vi "GermanInfo_settings_ut_test.vi"(8 "Error In":errorcluster, 11 "CSMinfo in":T1 {"Окно с настройками"."scheme" items=["NORMAL", "NORMAL_IMMEDIATE_START", "TIMEOUT_T3", "ALLRV_REQ", "SUPPRESS_MSD", "SUPPRESS_ALACK", "SUPPRESS_SEND_MSD"]}) -> (0 "Error Out":errorcluster, 3 "CSMinfo out":T1 {"Окно с настройками"."scheme" items=["NORMAL", "NORMAL_IMMEDIATE_START", "TIMEOUT_T3", "ALLRV_REQ", "SUPPRESS_MSD", "SUPPRESS_ALACK", "SUPPRESS_SEND_MSD"]})   [LabVIEW 2018]
uses:
  MOKO_LabViewLibrary/MokoSTM/MokoClassicUtilitySTM/MCUS_ITEM.ctl
  MOKO_LabViewLibrary/MokoSTM/MokoClassicUtilitySTM/MCUS_STM.ctl
  <vilib>/addons/_JKI.lib/Serialization/JSON/JKI JSON Serialization.lvlib
  GermanInfo.ctl
panel:
  in  "Input attenuation 5":dbl=1.0
  in  "Input attenuation 4":dbl=1.0
  in  "Input attenuation 3":dbl=1.0
  in  "Reset":bool
  in  "Open":bool
  in  "Save":bool
  in  "Setting Path":path
  in  "Применить":bool
  in  "Input attenuation 2":dbl=1.0
  in  "Режим звонка связь":u16(ring) items=["Автоматически (AT) GEMALTO", "Автоматически (AT) SIMCOM", "Автоматически (AT) SIMCOM SIM7600E-H", "Автоматически (AT) TELIT", "Автоматически (AT) PROGRESS", "Автоматически (AT) PROGRESS GREEN", "Автоматически (AT) PROGRESS BLUE", "Автоматически (реле)", "Вручную"]
  # "Входное напряжение (Uin_PS):"
  # "Входной ток (Iin_PS):"
  # "0,4\n0,6\n1\n1,5\n1,6\n2,5\n4"
  # "kPa\nbar\nkgf/cm2\nMPa"
  # "Выходное напряжение (Uout_EL):"
  # "Выходной ток (Iout_EL):"
  # "Схема измерений:"
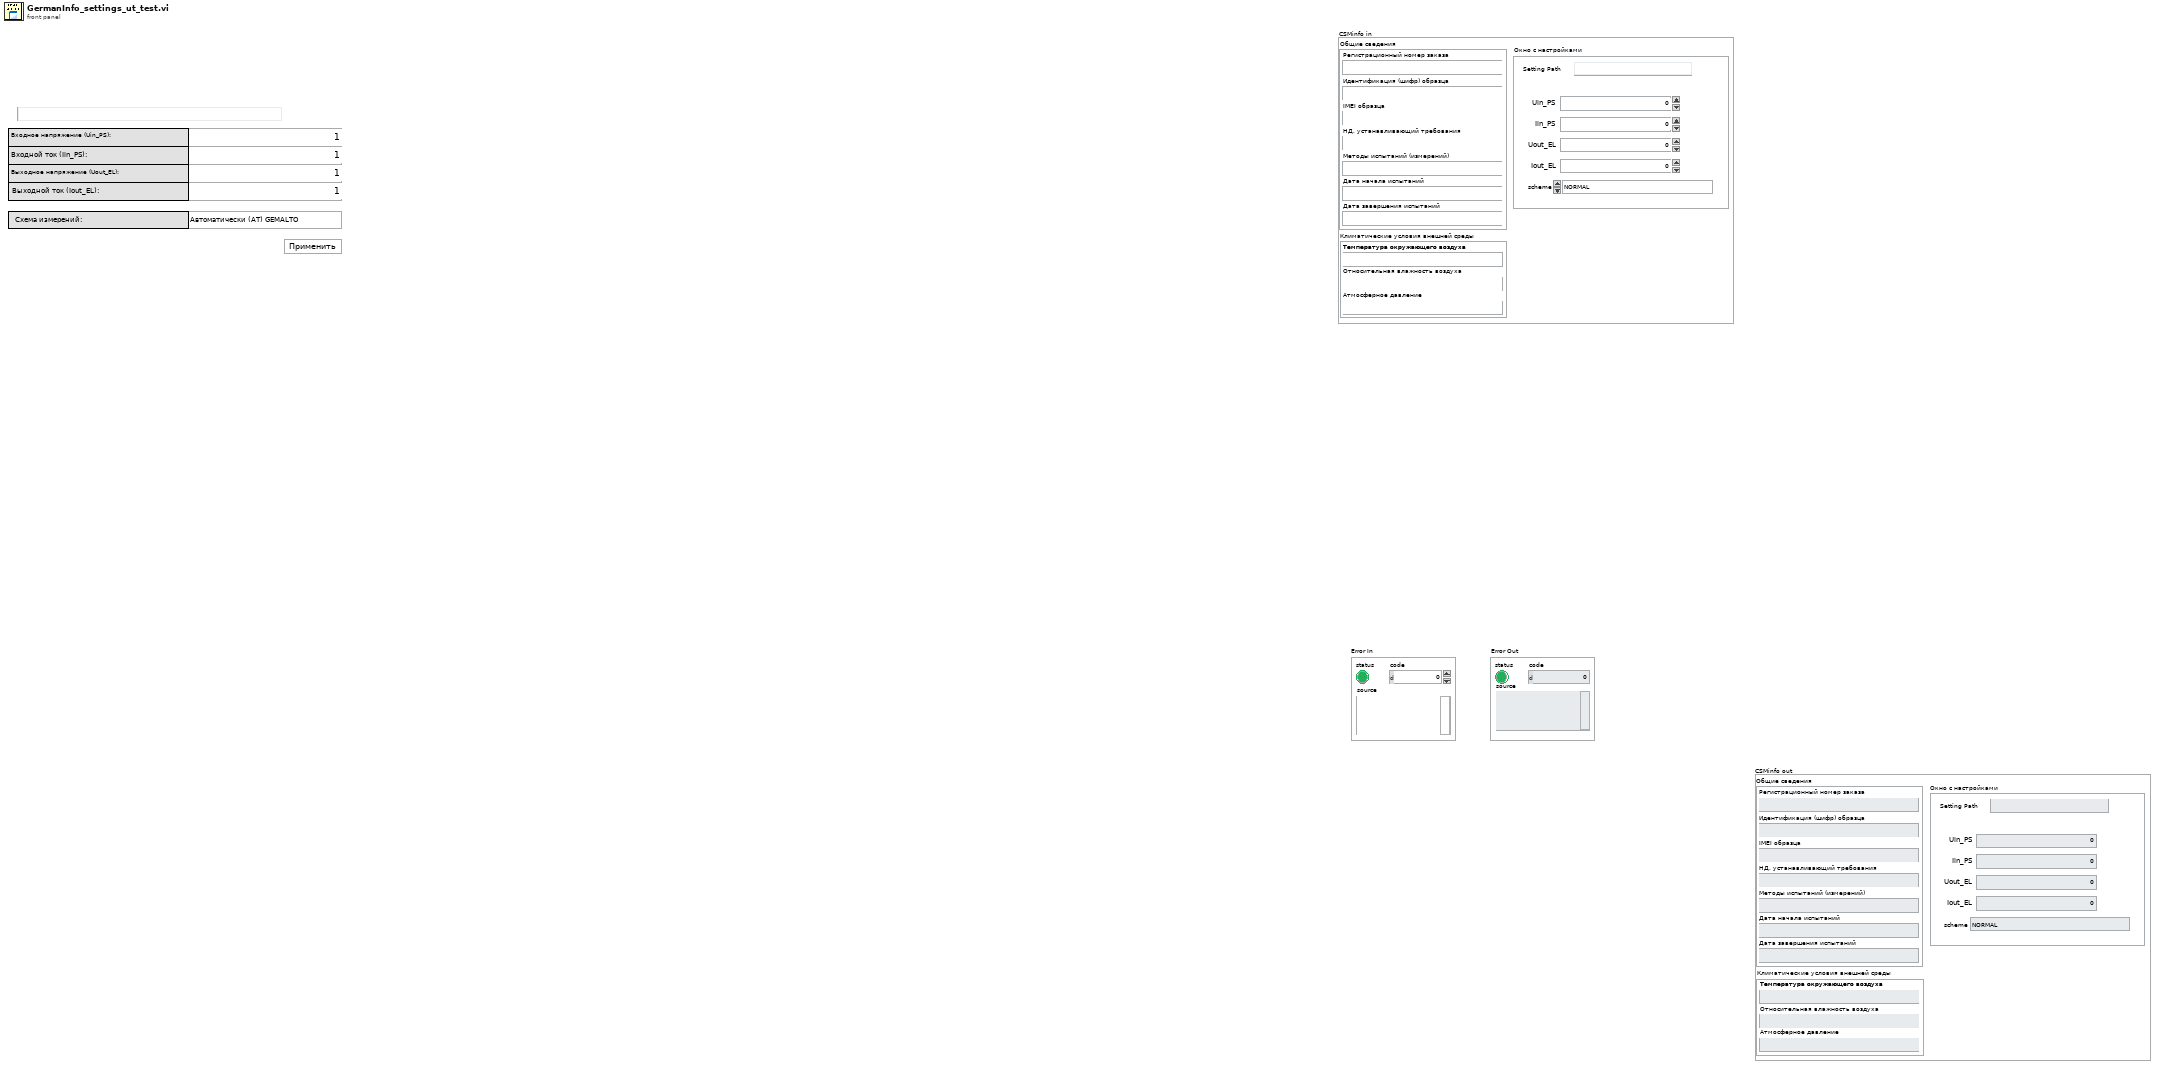
[diagram p1: front panel]
types:
  T1 = typedef "GermanInfo.ctl" = cluster{"Общие сведения":cluster{"Регистрационный номер заказа":string, "Идентификация (шифр) образца":string, "IMEI образца":string, "НД, устанавливающий требования":string, "Методы испытаний (измерений)":string, "Дата начала испытаний":string, "Дата завершения испытаний":string}, "Климатические условия внешней среды":cluster{"Температура окружающего воздуха":string, "Относительная влажность воздуха":string, "Атмосферное давление":string}, "Окно с настройками":cluster{"Uin_PS":dbl, "Setting Path":path, "Iin_PS":dbl, "Uout_EL":dbl, "Iout_EL":dbl, "scheme":u16}}
  T2 = typedef "MCUS_STM.ctl" = cluster{"main stm":T3, "data":string}
  T3 = typedef "MCUS_ITEM.ctl" = enum16{"idle", "_____ main_____ ", "Init", "Stop", "Apply values", "Save", "Open", "Reset"}
  T4 = cluster{"Uin_PS":dbl, "Setting Path":path, "Iin_PS":dbl, "Uout_EL":dbl, "Iout_EL":dbl, "scheme":u16}
  T5 = enum16{"open", "replace", "create", "open or create", "replace or create", "replace or create with confirmation"}
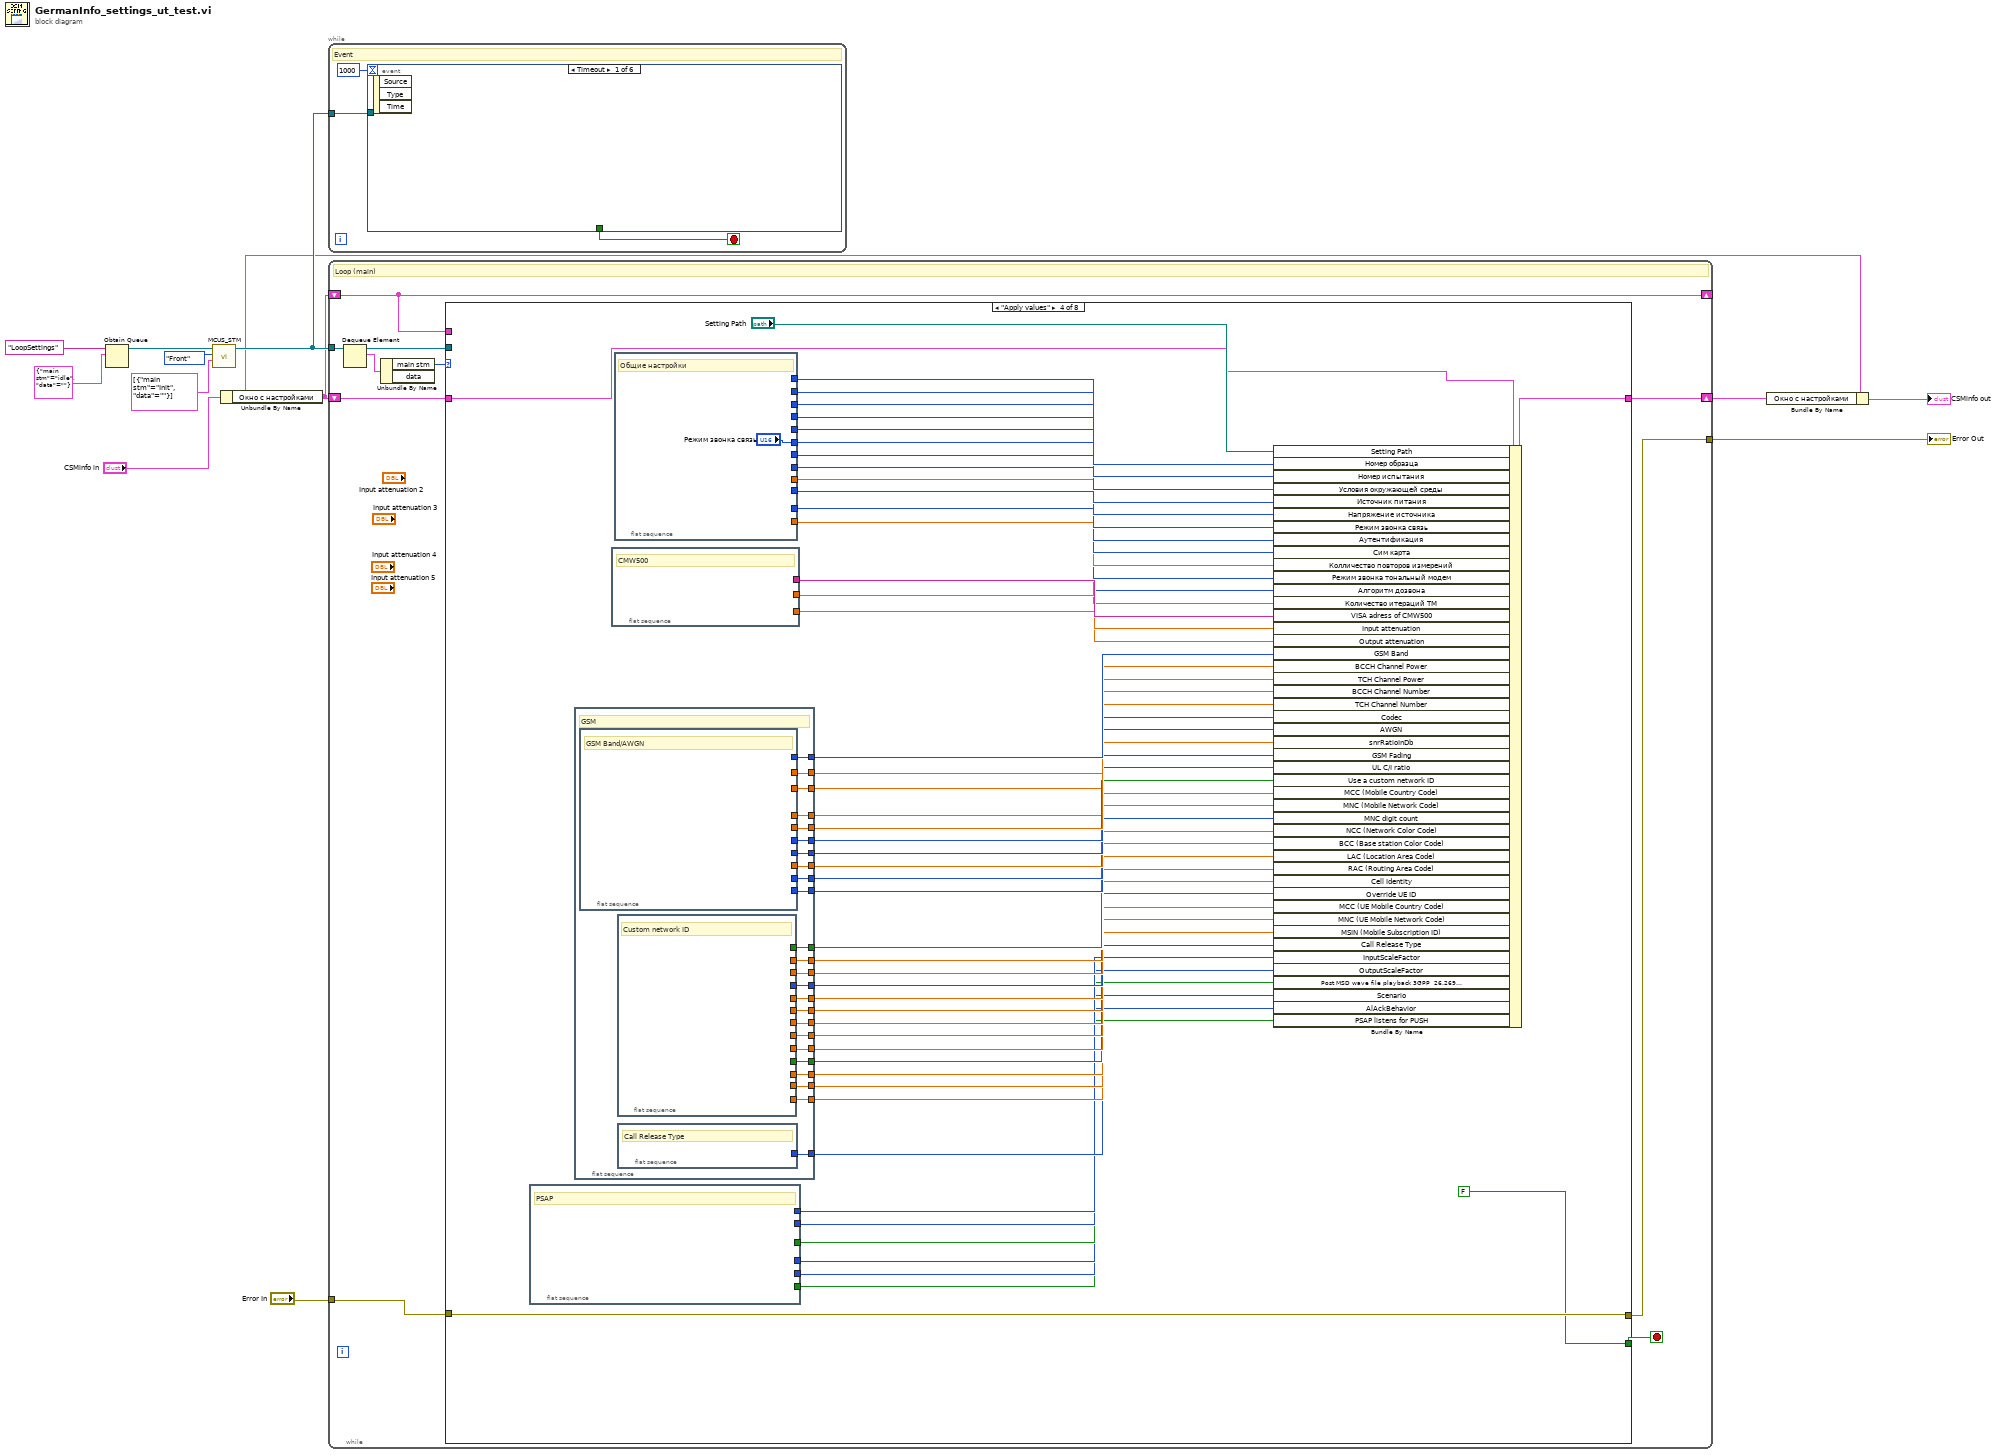
[diagram p0: block diagram]
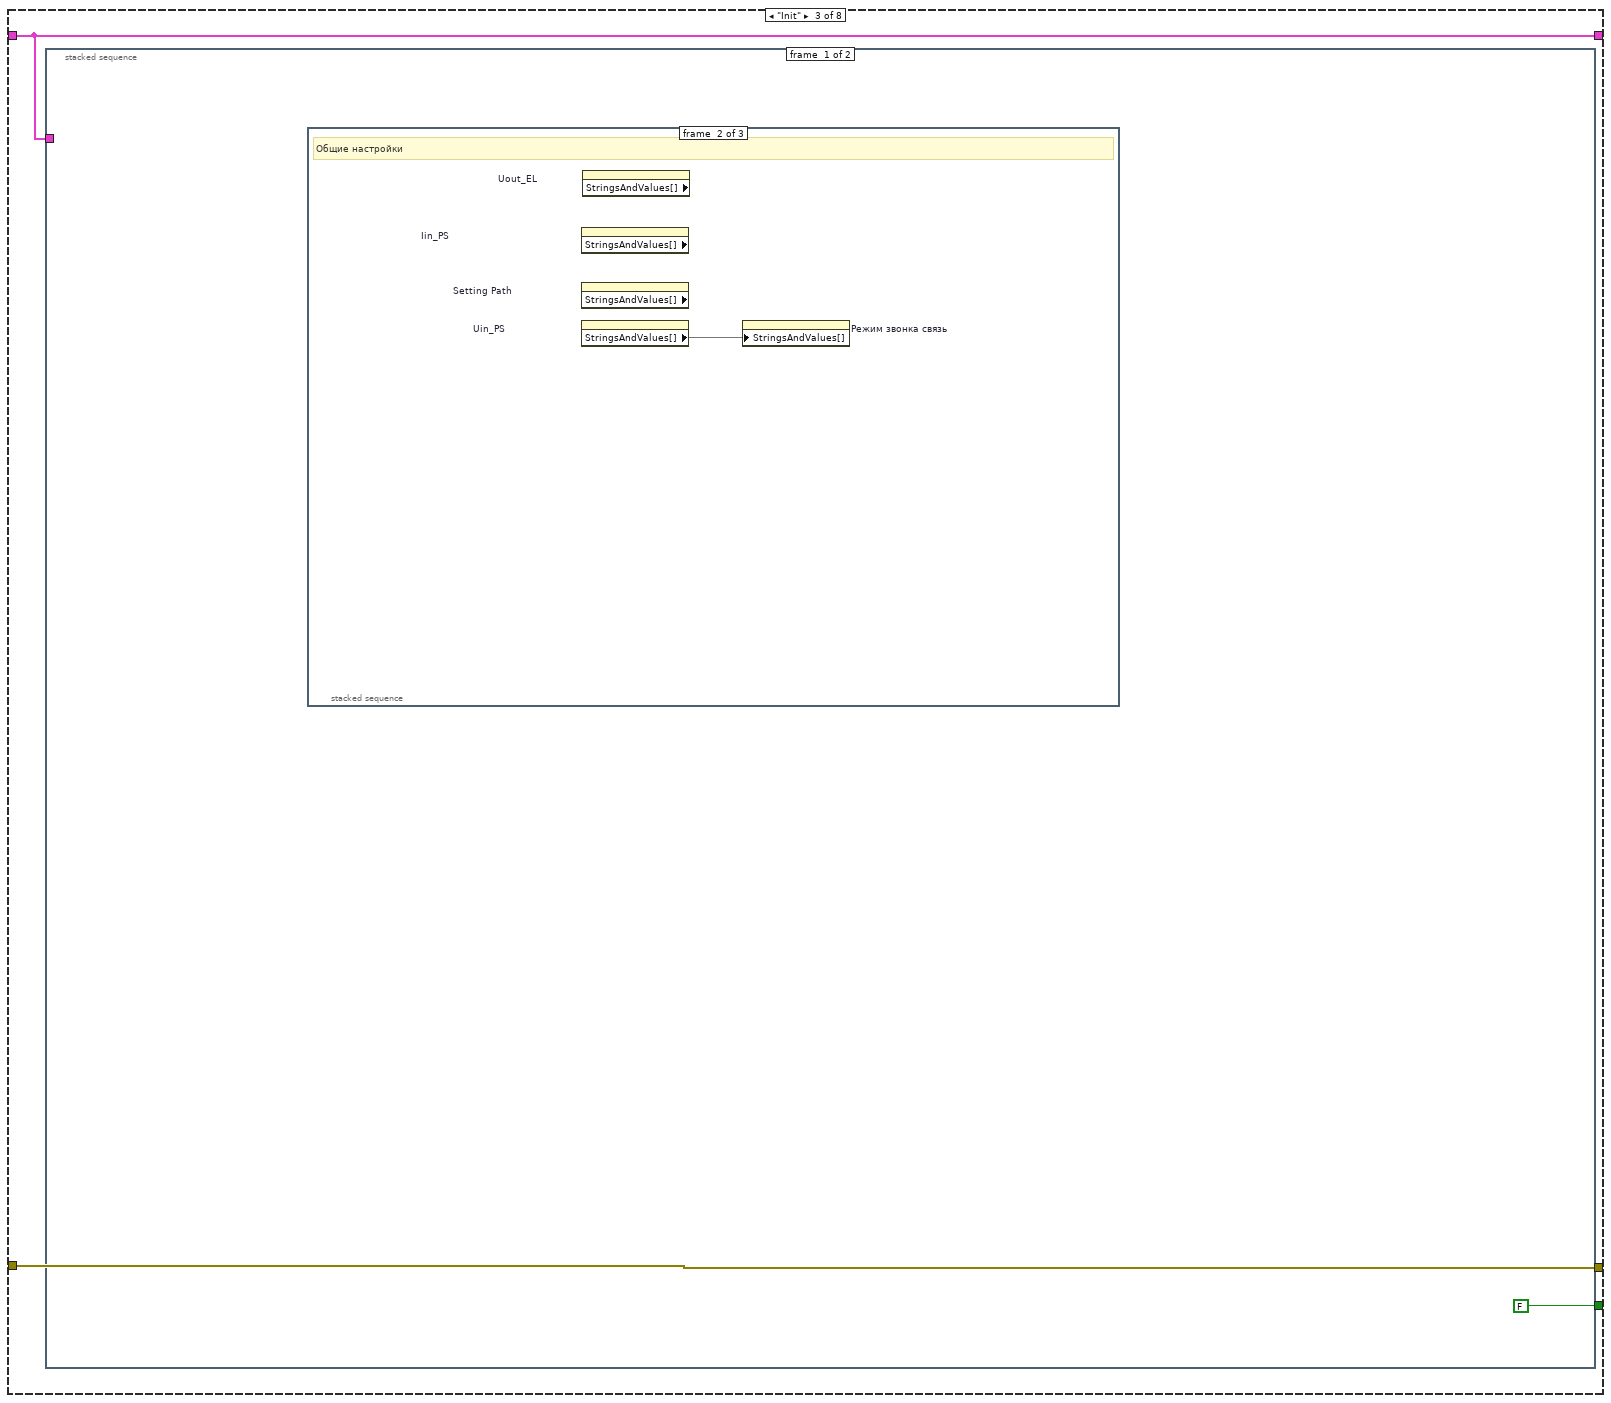
[diagram p4: hidden frame]
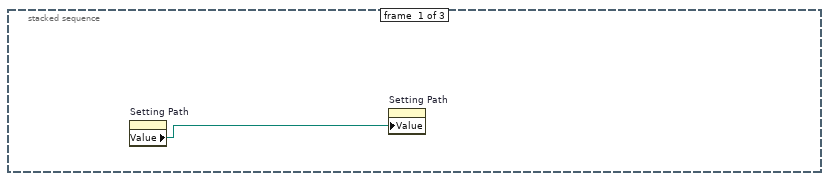
[diagram p5: hidden frame]
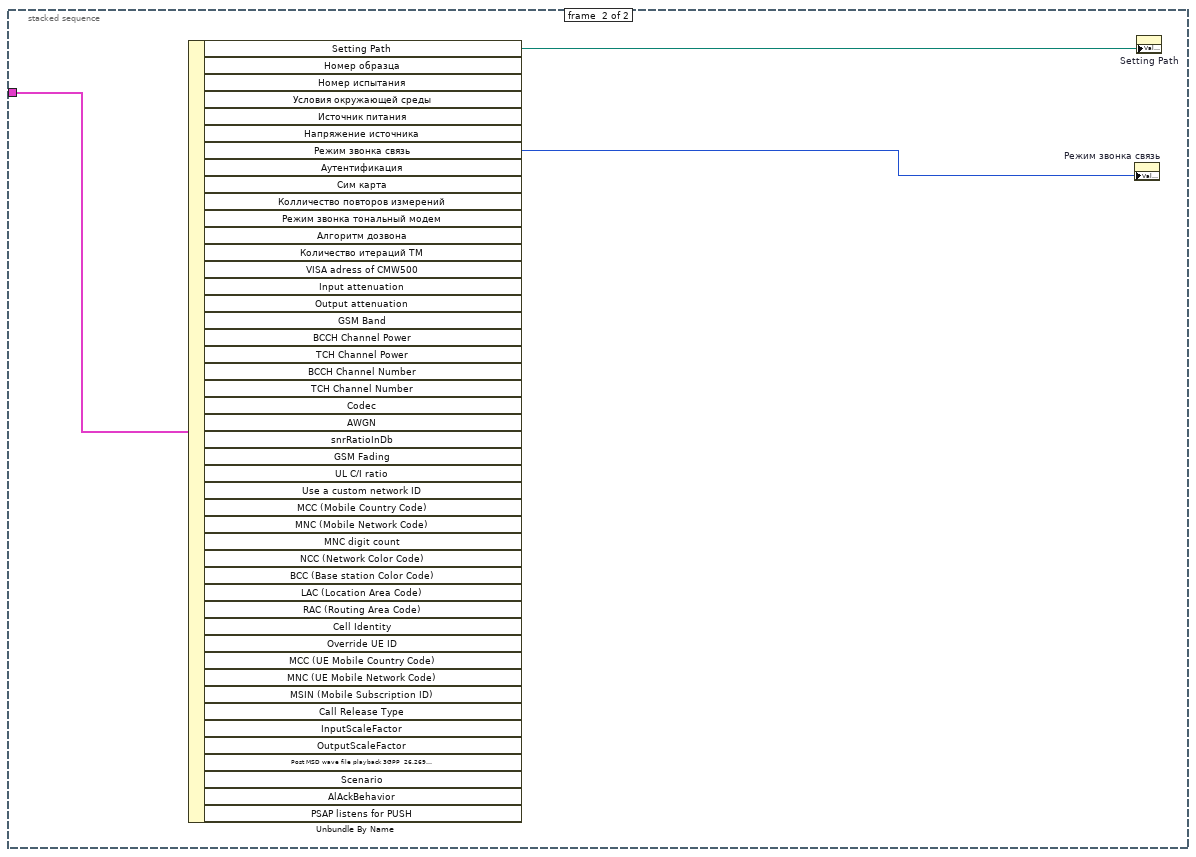
[diagram p11: hidden frame]
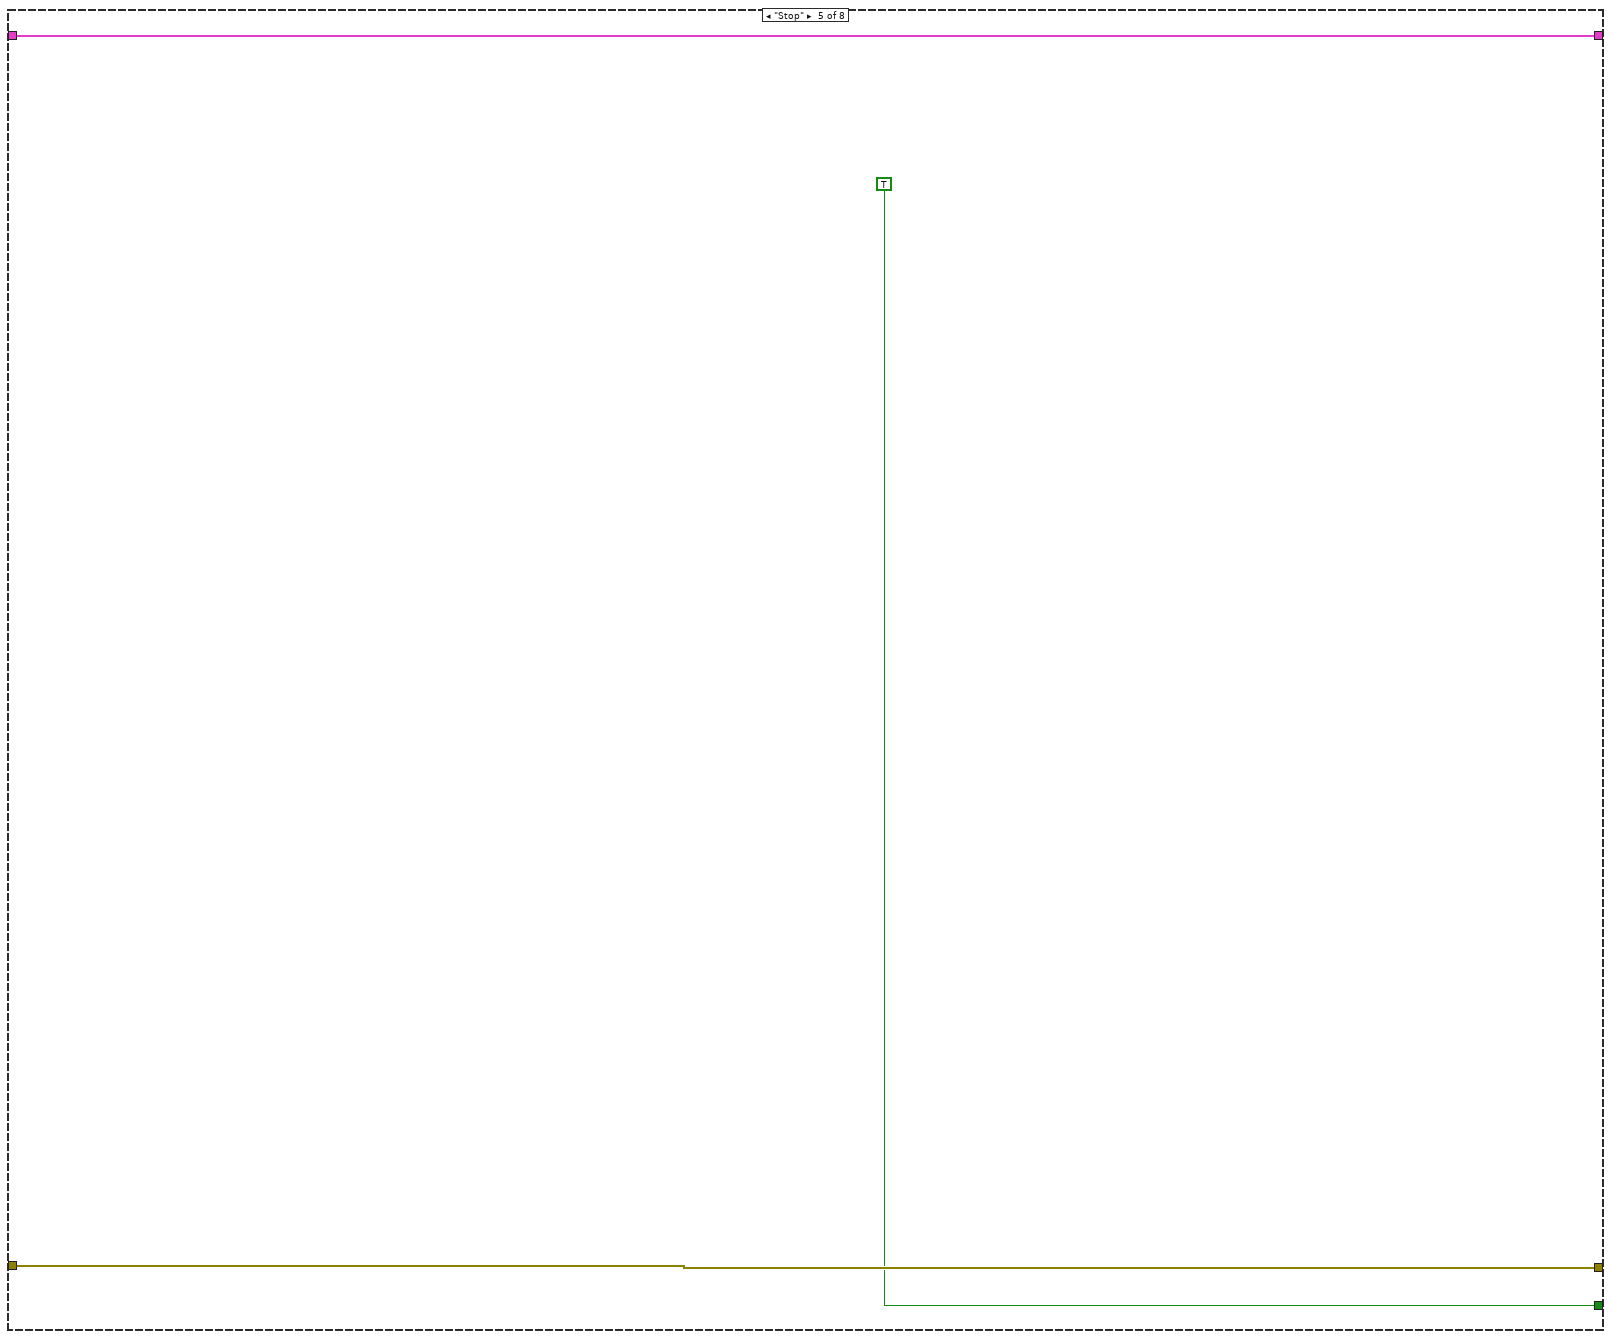
[diagram p12: hidden frame]
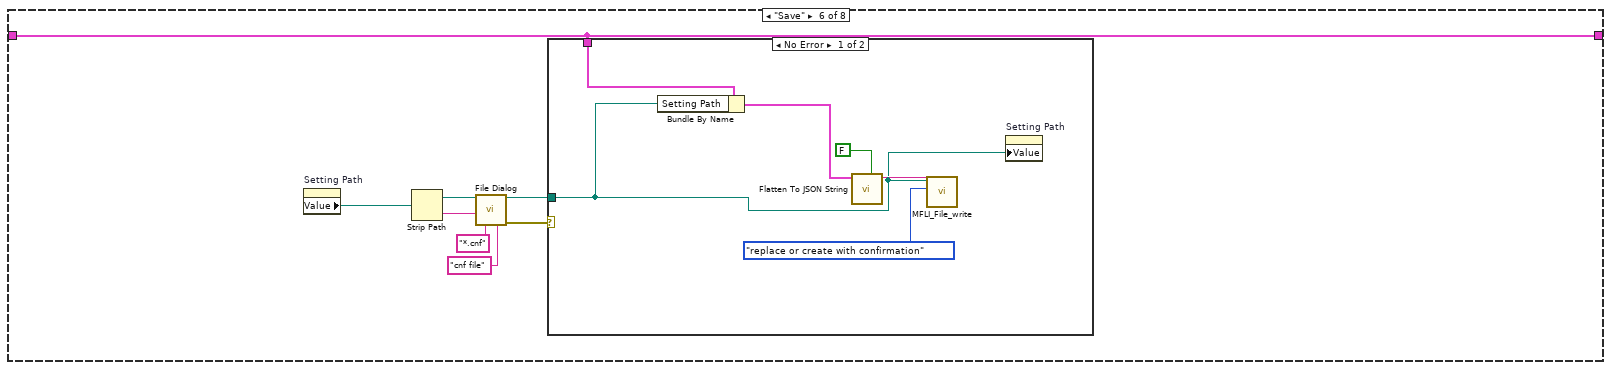
[diagram p13: hidden frame]
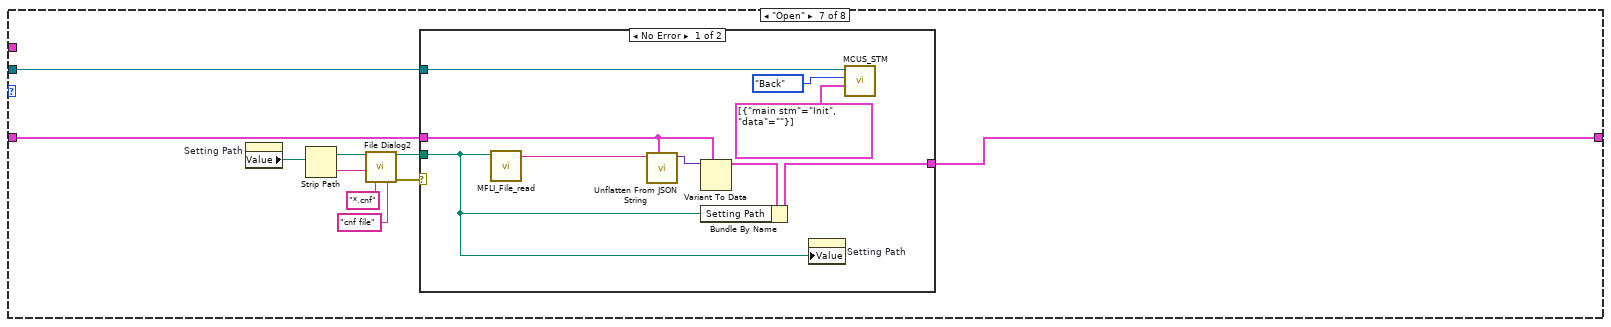
[diagram p15: hidden frame]
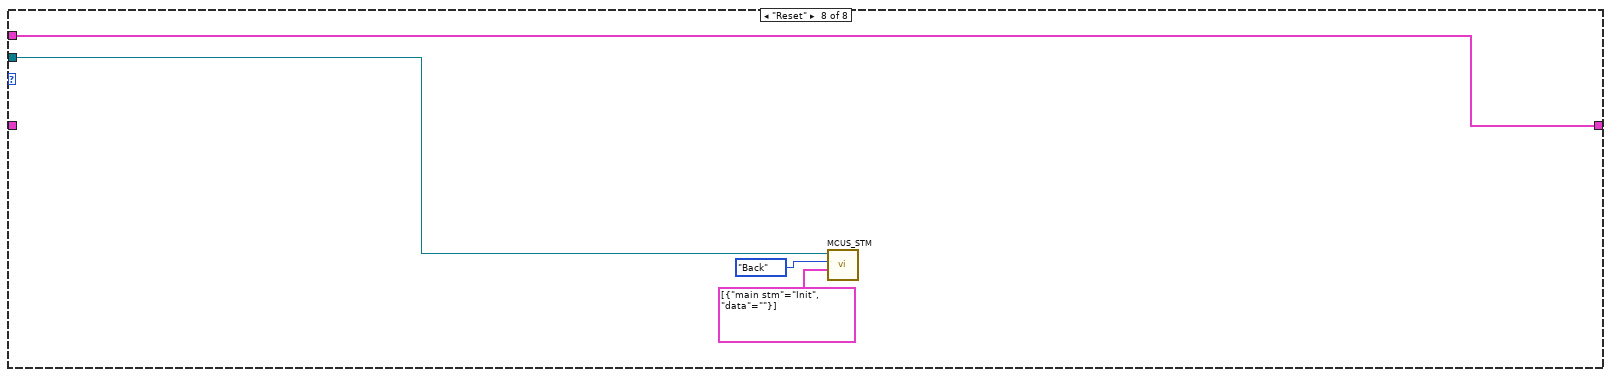
[diagram p17: hidden frame]
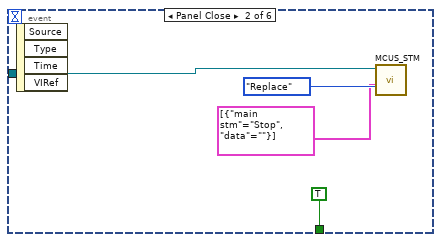
[diagram p18: hidden frame]
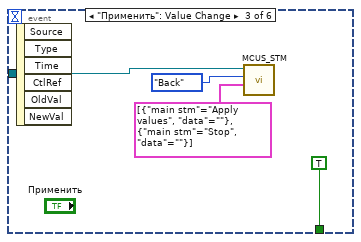
[diagram p19: hidden frame]
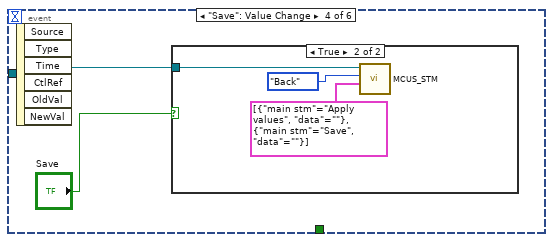
[diagram p20: hidden frame]
diagram:
  n1 = Obtain Queue(name (unnamed)="LoopSettings", element data type=T2 {"main stm"=enum."idle", "data"=""} ("MOKO_NMEA")) -> (queue out=w12:refnum<queue>)  [unwired: 3 in, 2 out]
  n2 = call "MCUS_STM.vi"("StateMachineSteps"=T2[] [{"main stm"=enum."Init", "data"=""}], "FNs"=enum16{"Back", "Front", "Replace"}."Front", "Queue in"=w12) -> ("Queue out"=w7:refnum<queue>)  [unwired: 7 in, 1 out]
  n3 = Unbundle By Name("CSMinfo in") -> ("Окно с настройками"=w4:T4)
  n4 = while {
    tunnel: w7 -> [w13]
    stop <- w15 stop-if-true
    # "Event"
    n5 = event shown="[0] Timeout" {
      selector: _ -> [_ _ _ _ _ _]
      dyn-events: _ -> [_ _ _ _ _ _]
      timeout: 1000 -> [_ _ _ _ _ _]
      tunnel: [_ TRUE TRUE _ _ _] -> w15
      tunnel: w13 -> [_ w16 w21 w25 w30 w35]
      event Timeout {
        n6 = event-data() -> ()  [unwired: 1 in, 3 out]
      }
      event Panel Close {
        n7 = event-data() -> ()  [unwired: 1 in, 4 out]
        n8 = call "MCUS_STM.vi"("StateMachineSteps"=T2[] [{"main stm"=enum."Stop", "data"=""}], "FNs"=enum16{"Back", "Front", "Replace"}."Replace", "Queue in"=w16) -> ()  [unwired: 7 in, 2 out]
      }
      event "Применить": Value Change {
        n9 = event-data() -> ()  [unwired: 1 in, 6 out]
        n10 = call "MCUS_STM.vi"("StateMachineSteps"=T2[] [{"main stm"=enum."Apply values", "data"=""}, {"main stm"=enum."Stop", "data"=""}], "FNs"=enum16{"Back", "Front", "Replace"}."Back", "Queue in"=w21) -> ()  [unwired: 7 in, 2 out]
      }
      event "Save": Value Change {
        n11 = event-data() -> ()  [unwired: 1 in, 6 out]
        n12 = case shown="True" "Save" {
          tunnel: w25 -> [_ w26]
          frame False {
          }
          frame True {
            n13 = call "MCUS_STM.vi"("StateMachineSteps"=T2[] [{"main stm"=enum."Apply values", "data"=""}, {"main stm"=enum."Save", "data"=""}], "FNs"=enum16{"Back", "Front", "Replace"}."Back", "Queue in"=w26) -> ()  [unwired: 7 in, 2 out]
          }
        }
      }
      event "Open": Value Change {
        n14 = event-data() -> ()  [unwired: 1 in, 6 out]
        n15 = case shown="True" "Open" {
          tunnel: w30 -> [_ w31]
          frame False {
          }
          frame True {
            n16 = call "MCUS_STM.vi"("StateMachineSteps"=T2[] [{"main stm"=enum."Open", "data"=""}], "FNs"=enum16{"Back", "Front", "Replace"}."Back", "Queue in"=w31) -> ()  [unwired: 7 in, 2 out]
          }
        }
      }
      event "Reset": Value Change {
        n17 = event-data() -> ()  [unwired: 1 in, 6 out]
        n18 = case shown="True" "Reset" {
          tunnel: w35 -> [_ w36]
          frame False {
          }
          frame True {
            n19 = call "MCUS_STM.vi"("StateMachineSteps"=T2[] [{"main stm"=enum."Reset", "data"=""}], "FNs"=enum16{"Back", "Front", "Replace"}."Back", "Queue in"=w36) -> ()  [unwired: 7 in, 2 out]
          }
        }
      }
    }
  }
  n20 = while {
    tunnel: w7 -> [w48]
    tunnel: "Error In" -> [w44]
    tunnel: [w43] -> w5
    shift-right: [w42] -> w2
    shift-left: w4 -> [w40]
    shift-right: [w39] -> _
    shift-left: w4 -> [w39]
    stop <- w45 stop-if-true
    # "Loop (main)"
    n21 = Dequeue Element(queue=w48) -> (queue out=w41:refnum<queue>, element=w47:T2)  [unwired: 2 in, 2 out]
    n22 = Unbundle By Name(w47) -> ("main stm"=w46:T3)  [unwired: 1 out]
    n23 = case shown="\"Apply values\"" w46 {
      tunnel: w41 -> [_ _ _ _ _ _ w234 w251]
      tunnel: [_ _ FALSE FALSE TRUE _ _ _] -> w45
      tunnel: w44 -> [w50 w52 w55 w157 w216 _ _ _]
      tunnel: [w50 w52 w55 w157 w216 _ _ _] -> w43
      tunnel: [w49 w51 w53 w155 w214 w220 w236 w254] -> w42
      tunnel: w40 -> [w49 w51 w53 w109 w214 w220 w235 _]
      tunnel: w39 -> [_ _ _ _ _ _ _ w254]
      frame "idle", Default {
      }
      frame "_____ main_____ " {
      }
      frame "Init" {
        n24 = stacked-sequence {
          tunnel: w53 -> [_ w107]
          frame #0 {
            n25 = stacked-sequence {
              frame #0 {
                n26 = property on="Setting Path" class="Path"() -> ("Value"=w56:path)  [unwired: 2 in, 2 out]
                n27 = property on="Setting Path" class="Path"("Value"=w56) -> ()  [unwired: 2 in, 2 out]
              }
              frame #1 {
                # "Общие настройки"
                n28 = property on="Iin_PS" class="DigNum (strict)"() -> ("StringsAndValues[]"=w60)  [unwired: 2 in, 2 out]
                n29 = property on="Setting Path" class="Path"() -> ("StringsAndValues[]"=w59)  [unwired: 2 in, 2 out]
                n30 = property on="Uin_PS" class="DigNum (strict)"() -> ("StringsAndValues[]"=w57)  [unwired: 2 in, 2 out]
                n31 = property on="Uout_EL" class="DigNum (strict)"() -> ("StringsAndValues[]"=w58)  [unwired: 2 in, 2 out]
                n32 = property on="Режим звонка связь" class="Ring (strict)"("StringsAndValues[]"=w57) -> ()  [unwired: 2 in, 2 out]
              }
              frame #2 {
                # "Настройки модема по умолчанию"
                n33 = stacked-sequence {
                  frame #0 {
                    # "CMW500"
                  }
                  frame #1 {
                    # "GSM"
                    n34 = stacked-sequence {
                      frame #0 {
                        # "GSM Band/AWGN"
                      }
                      frame #1 {
                        # "Custom network ID"
                      }
                      frame #2 {
                        # "Call Release Type"
                      }
                    }
                  }
                  frame #2 {
                    # "PSAP"
                  }
                }
              }
            }
          }
          frame #1 {
            n35 = Unbundle By Name(w107) -> ("Setting Path"=w63:path, "Номер образца"=w106:u16, "Номер испытания"=w105:u16, "Условия окружающей среды"=w104:u16, "Источник питания"=w103:u16, "Напряжение источника"=w102:u16, "Режим звонка связь"=w101:u16, "Аутентификация"=w98:u16, "Сим карта"=w96:u16, "Колличество повторов измерений"=w97:dbl, "Режим звонка тональный модем"=w100:u16, "Алгоритм дозвона"=w61:u16, "Количество итераций TM"=w99:dbl, "VISA adress of CMW500"=w95:string, "Input attenuation"=w94:dbl, "Output attenuation"=w93:dbl, "GSM Band"=w92:u16, "BCCH Channel Power"=w65:dbl, "TCH Channel Power"=w64:dbl, "BCCH Channel Number"=w62:dbl, "TCH Channel Number"=w91:dbl, "Codec"=w90:u16, "AWGN"=w89:u16, "snrRatioInDb"=w88:dbl, "GSM Fading"=w87:u16, "UL C/I ratio"=w86:u16, "Use a custom network ID"=w85:bool, "MCC (Mobile Country Code)"=w84:dbl, "MNC (Mobile Network Code)"=w83:dbl, "MNC digit count"=w82:u16, "NCC (Network Color Code)"=w81:dbl, "BCC (Base station Color Code)"=w80:dbl, "LAC (Location Area Code)"=w79:dbl, "RAC (Routing Area Code)"=w78:dbl, "Cell Identity"=w77:dbl, "Override UE ID"=w76:bool, "MCC (UE Mobile Country Code)"=w75:dbl, "MNC (UE Mobile Network Code)"=w74:dbl, "MSIN (Mobile Subscription ID)"=w73:dbl, "Call Release Type"=w72:u16, "InputScaleFactor"=w71:u16, "OutputScaleFactor"=w70:u16, "Post MSD wave file playback 3GPP  26.269 \nEU_DTMF_tones"=w69:bool, "Scenario"=w68:u16, "AlAckBehavior"=w67:u16, "PSAP listens for PUSH"=w66:bool)
            n36 = property on="Режим звонка связь" class="Ring (strict)"("Value"=w101) -> ()  [unwired: 2 in, 2 out]
            n37 = property on="Setting Path" class="Path"("Value"=w63) -> ()  [unwired: 2 in, 2 out]
          }
        }
      }
      frame "Apply values" {
        n38 = flat-sequence {
          tunnel: [_] -> w119
          tunnel: [_] -> w118
          tunnel: [_] -> w117
          tunnel: [_] -> w116
          tunnel: [_] -> w115
          tunnel: [_] -> w114
          frame #0 {
            # "PSAP"
          }
        }
        n39 = flat-sequence {
          tunnel: [w181] -> w140
          tunnel: [w180] -> w113
          tunnel: [w179] -> w139
          tunnel: [w178] -> w138
          tunnel: [w177] -> w137
          tunnel: [w176] -> w136
          tunnel: [w175] -> w135
          tunnel: [w174] -> w134
          tunnel: [w173] -> w133
          tunnel: [w172] -> w132
          tunnel: [w171] -> w131
          tunnel: [w170] -> w130
          tunnel: [w169] -> w129
          tunnel: [w168] -> w128
          tunnel: [w167] -> w127
          tunnel: [w166] -> w126
          tunnel: [w165] -> w125
          tunnel: [w164] -> w124
          tunnel: [w163] -> w123
          tunnel: [w162] -> w122
          tunnel: [w161] -> w121
          tunnel: [w160] -> w120
          tunnel: [w159] -> w112
          tunnel: [w158] -> w111
          frame #0 {
            # "GSM"
            n40 = flat-sequence {
              tunnel: [w205] -> w181
              tunnel: [w204] -> w180
              tunnel: [w203] -> w179
              tunnel: [w202] -> w178
              tunnel: [w201] -> w177
              tunnel: [w200] -> w176
              tunnel: [w199] -> w175
              tunnel: [w198] -> w174
              tunnel: [w197] -> w159
              tunnel: [w196] -> w158
              frame #0 {
                # "GSM Band/AWGN"
              }
            }
            n41 = flat-sequence {
              tunnel: [w195] -> w173
              tunnel: [w194] -> w172
              tunnel: [w193] -> w171
              tunnel: [w192] -> w170
              tunnel: [w191] -> w169
              tunnel: [w190] -> w168
              tunnel: [w189] -> w167
              tunnel: [w188] -> w166
              tunnel: [w187] -> w165
              tunnel: [w186] -> w164
              tunnel: [w185] -> w163
              tunnel: [w184] -> w162
              tunnel: [w183] -> w161
              frame #0 {
                # "Custom network ID"
              }
            }
            n42 = flat-sequence {
              tunnel: [w182] -> w160
              frame #0 {
                # "Call Release Type"
              }
            }
          }
        }
        n43 = flat-sequence {
          tunnel: [w213] -> w146
          tunnel: [w212] -> w145
          tunnel: [w211] -> w144
          frame #0 {
            # "CMW500"
          }
        }
        n44 = flat-sequence {
          tunnel: [w210] -> w154
          tunnel: [_] -> w153
          tunnel: [_] -> w152
          tunnel: [_] -> w151
          tunnel: [_] -> w150
          tunnel: ["Режим звонка связь"] -> w149
          tunnel: [_] -> w148
          tunnel: [w208] -> w147
          tunnel: [_] -> w143
          tunnel: [_] -> w142
          tunnel: [w207] -> w141
          tunnel: [w206] -> w108
          frame #0 {
            # "Общие настройки"
          }
        }
        n45 = Bundle By Name(cluster=w109, "Setting Path"="Setting Path", "Номер образца"=w154, "Номер испытания"=w153, "Условия окружающей среды"=w152, "Источник питания"=w151, "Напряжение источника"=w150, "Режим звонка связь"=w149, "Аутентификация"=w148, "Сим карта"=w147, "Колличество повторов измерений"=w143, "Режим звонка тональный модем"=w142, "Алгоритм дозвона"=w108, "Количество итераций TM"=w141, "VISA adress of CMW500"=w146, "Input attenuation"=w145, "Output attenuation"=w144, "GSM Band"=w140, "BCCH Channel Power"=w112, "TCH Channel Power"=w111, "BCCH Channel Number"=w113, "TCH Channel Number"=w139, "Codec"=w138, "AWGN"=w137, "snrRatioInDb"=w136, "GSM Fading"=w135, "UL C/I ratio"=w134, "Use a custom network ID"=w133, "MCC (Mobile Country Code)"=w132, "MNC (Mobile Network Code)"=w131, "MNC digit count"=w130, "NCC (Network Color Code)"=w129, "BCC (Base station Color Code)"=w128, "LAC (Location Area Code)"=w127, "RAC (Routing Area Code)"=w126, "Cell Identity"=w125, "Override UE ID"=w124, "MCC (UE Mobile Country Code)"=w123, "MNC (UE Mobile Network Code)"=w122, "MSIN (Mobile Subscription ID)"=w121, "Call Release Type"=w120, "InputScaleFactor"=w119, "OutputScaleFactor"=w118, "Post MSD wave file playback 3GPP  26.269 \nEU_DTMF_tones"=w117, "Scenario"=w116, "AlAckBehavior"=w115, "PSAP listens for PUSH"=w114) -> (w155:T4)
      }
      frame "Stop" {
      }
      frame "Save" {
        n46 = property on="Setting Path" class="Path"() -> ("Value"=w219:path)  [unwired: 2 in, 2 out]
        n47 = Strip Path(path=w219) -> (stripped path=w218:path, name=w217:string)
        n48 = call "File Dialog"("start path"=w218, "default name"=w217, "pattern (all files)"="*.cnf", "pattern label"="cnf file") -> ("selected path"=w222:path, "error out"=w221:errorcluster)  [unwired: 8 in, 2 out]
        n49 = case shown="No Error" w221 {
          tunnel: w220 -> [w227 _]
          tunnel: w222 -> [w226 _]
          frame No Error {
            n50 = Bundle By Name(cluster=w227, "Setting Path"=w226) -> (w225:T4)
            n51 = call <vilib>:"Flatten To JSON String.vi"("Numeric Extensions (F)"=FALSE, "Variant"=w225) -> ("JSON String"=w229:string)  [unwired: 8 in, 1 out]
            n52 = call "MFLI_File_write.vi"("String"=w229, "operation (0:open)"=T5."replace or create with confirmation", "selected path"=w226) -> ()  [unwired: 7 in, 2 out]
            n53 = property on="Setting Path" class="Path"("Value"=w226) -> ()  [unwired: 2 in, 2 out]
          }
          frame Error {
          }
        }
      }
      frame "Open" {
        n54 = property on="Setting Path" class="Path"() -> ("Value"=w233:path)  [unwired: 2 in, 2 out]
        n55 = Strip Path(path=w233) -> (stripped path=w231:path, name=w232:string)
        n56 = call "File Dialog2"("start path"=w231, "default name"=w232, "pattern (all files)"="*.cnf", "pattern label"="cnf file") -> ("selected path"=w238:path, "error out"=w237:errorcluster)  [unwired: 8 in, 2 out]
        n57 = case shown="No Error" w237 {
          tunnel: w238 -> [w241 _]
          tunnel: w234 -> [w247 _]
          tunnel: w235 -> [w245 w250]
          tunnel: [w242 w250] -> w236
          frame No Error {
            n58 = call "MFLI_File_read.vi"("Project script or program"=w241) -> ("String"=w246:string)  [unwired: 9 in, 1 out]
            n59 = call <vilib>:"Unflatten From JSON String.vi"("Type and Defaults"=w245, "JSON String"=w246) -> ("Variant"=w244:variant)  [unwired: 8 in, 1 out]
            n60 = Variant To Data(type=w245, Variant=w244) -> (data=w243:T4)  [unwired: 1 in, 1 out]
            n61 = Bundle By Name(cluster=w243, "Setting Path"=w241) -> (w242:T4)
            n62 = property on="Setting Path" class="Path"("Value"=w241) -> ()  [unwired: 2 in, 2 out]
            n63 = call "MCUS_STM.vi"("StateMachineSteps"=T2[] [{"main stm"=enum."Init", "data"=""}], "FNs"=enum16{"Back", "Front", "Replace"}."Back", "Queue in"=w247) -> ()  [unwired: 7 in, 2 out]
          }
          frame Error {
          }
        }
      }
      frame "Reset" {
        n64 = call "MCUS_STM.vi"("StateMachineSteps"=T2[] [{"main stm"=enum."Init", "data"=""}], "FNs"=enum16{"Back", "Front", "Replace"}."Back", "Queue in"=w251) -> ()  [unwired: 7 in, 2 out]
      }
    }
  }
  "Error Out" <- w5
  n65 = Bundle By Name(cluster="CSMinfo in", "Окно с настройками"=w2) -> (→"CSMinfo out":T1)
